vi "Sender.vi"() -> ()   [LabVIEW 2020]
uses:
  DataType.ctl
  <vilib>/ReMiSYS Technology/RemoteToolkit/Sender/Sender.lvclass
panel:
  in  "Value":T1 {"Tank 5" scale=0.0..255.0; "Tank 4" scale=0.0..255.0; "Tank 3" scale=0.0..255.0; "Tank 2" scale=0.0..255.0; "Tank" scale=0.0..255.0}
  in  "IP Address":string="127.0.0.1"
  out "Error Out":errorcluster
  in  "Stop":bool
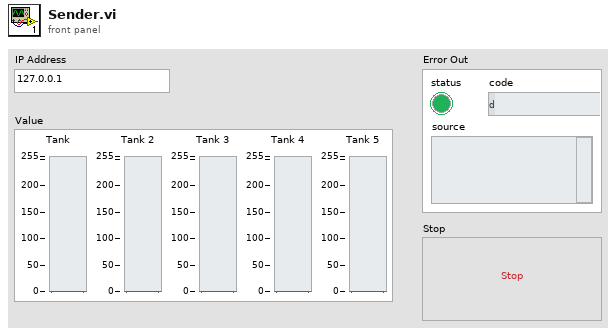
[diagram p1: front panel]
types:
  T1 = typedef "DataType.ctl" = cluster{"Tank":u8, "Tank 2":u8, "Tank 3":u8, "Tank 4":u8, "Tank 5":u8}
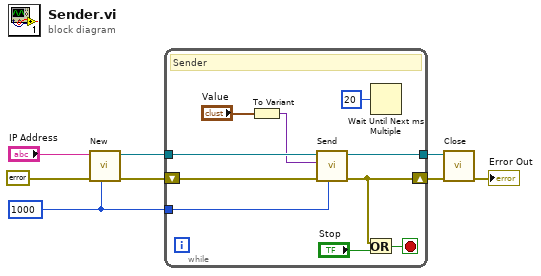
[diagram p0: block diagram]
diagram:
  w6 = 1000 ("Timeout ms (25000)")
  n1 = call <vilib>:"New.vi"("Timeout ms (25000)"=w6, "Error In"=errorcluster {"status"=FALSE, "code"=0, "source"=""}, "IP Address"="IP Address") -> ("Error Out"=w7:errorcluster, "Sender Ref."=w4:refnum<class "Sender.lvclass">)  [unwired: 7 in]
  n2 = while {
    shift-right: [w13] -> w3
    shift-left: w7 -> [w15]
    tunnel: w4 -> [w16]
    tunnel: w6 -> [w10]
    tunnel: [w14] -> w2
    stop <- w17 stop-if-true
    # "Sender"
    n3 = To Variant(anything="Value") -> (Variant=w11:variant)
    n4 = call <vilib>:"Send.vi"("Timeout ms (1000)"=w10, "Error In"=w15, "Value"=w11, "Sender Ref."=w16) -> ("Error Out"=w13:errorcluster, "Sender Ref."=w14:refnum<class "Sender.lvclass">)  [unwired: 6 in]
    n5 = Or(x=w13, y="Stop") -> (x .or. y?=w17:bool)
    n6 = Wait Until Next ms Multiple(millisecond multiple=u32 20) -> ()  [unwired: 1 out]
  }
  n7 = call <vilib>:"Close.vi"("Error In"=w3, "Receiver Ref."=w2) -> ("Error Out"=→"Error Out":errorcluster)  [unwired: 9 in]
